vi "VerySimpleCalibCheck.vi"() -> ()   [LabVIEW 2024]
uses:
  <vilib>/Analysis/5stat.llb/RMS (DBL).vi
  <vilib>/Analysis/NI_AALPro.lvlib
panel:
  in  "Gain":dbl=10.0
  in  "y":dbl=13.8
  out "mV/m/s2":dbl=74.80921598120463
  out "Volts":dbl=1.0578023139742336
  out "rms value":dbl=0.1713998464349972 format="%0.6f"
  out "peak":dbl=0.07665234159233576
  out "Data":dynamicdata(graph)=[{"t0"=timestamp(3623963203.341959 s since 1904-01-01), "dt"=2.2727272727272726e-05, "Y"=array[440 elements]}]
  # "Shoudl be 1 volt at 1 KHz"
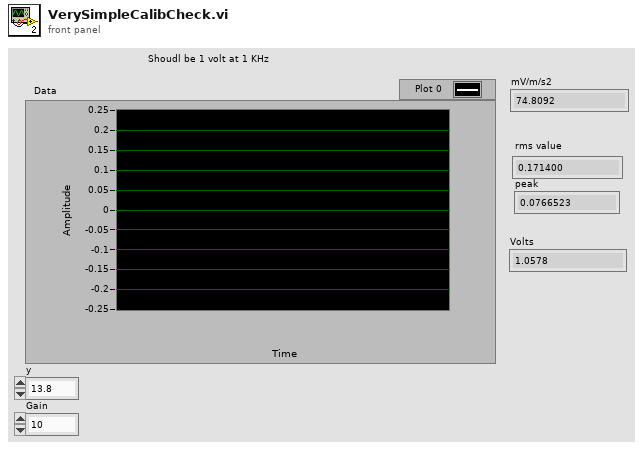
[diagram p1: front panel]
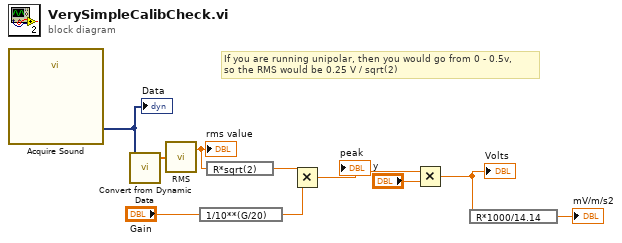
[diagram p0: block diagram]
diagram:
  # "If you are running unipolar, then you would go from 0 - 0.5v,\nso the RMS would be 0.25 V / sqrt(2)"
  n1 = call "Acquire Sound"() -> ("Data"=w9:dynamicdata)  [unwired: 18 in, 1 out]
  "Data" <- w9
  n2 = call "Convert from Dynamic Data"("Dynamic Data Type"=w9) -> ("Array"=w8:dbl[])  [unwired: 3 in]
  n3 = call-poly <vilib>:"RMS.vi"("X"=w8) -> ("rms value"=w10:dbl)  [unwired: 1 out]
  "rms value" <- w10
  n4 = expression code="1/10**(G/20)"("Gain") -> (w1:dbl)
  n5 = expression code="R*sqrt(2)"(w10) -> (w4:dbl)
  n6 = Multiply(x=w4, y=w1) -> (x*y=w3:dbl)
  "peak" <- w3
  n7 = Multiply(x=w3, y="y") -> (x*y=w5:dbl)
  "Volts" <- w5
  n8 = expression code="R*1000/14.14"(w5) -> (→"mV/m/s2":dbl)
